vi "Read Boolean Color Props.vi"(8 "error in (no error)":errorcluster, 11 "Control in":refnum<vi>) -> (0 "error out":errorcluster, 2 "Boolean Colors Props":T1, 3 "Control":refnum<vi>)   [LabVIEW 2020, in "VolatusGUIEditorCore.lvlib"]
uses:
  VolatusGUIEditorCore.lvlib
  Boolean Color Props.ctl
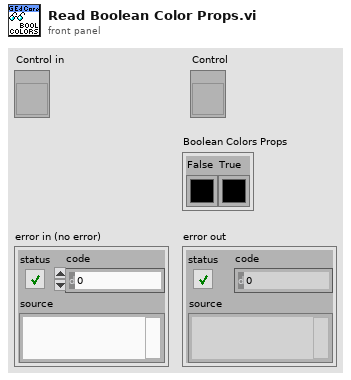
[diagram p1: front panel]
types:
  T1 = typedef "VolatusGUIEditorCore.lvlib/Boolean Color Props.ctl" = cluster{"False":u32, "True":u32}
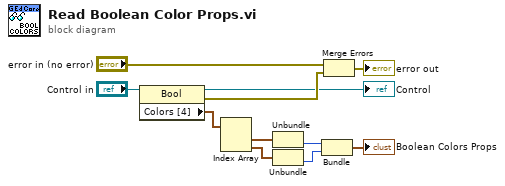
[diagram p0: block diagram]
diagram:
  n1 = property class="Bool"(reference="Control in") -> (reference out=→"Control":refnum<vi>, error out=w11:errorcluster, "Colors [4]"=w6:cluster{u32, u32}[])  [unwired: 1 in]
  n2 = Index Array(array=w6) -> (element #1=w5:cluster{u32, u32}, element #2=w4:cluster{u32, u32})  [unwired: 2 in]
  n3 = Unbundle(w5) -> (w2:u32)  [unwired: 1 out]
  n4 = Unbundle(w4) -> (w1:u32)  [unwired: 1 out]
  n5 = Bundle(w2, w1) -> (→"Boolean Colors Props":cluster{u32, u32})  [unwired: 1 in]
  n6 = Merge Errors("error in (no error)", w11) -> (→"error out":errorcluster)
